vi "Run and Terminate Servos Arduino --LINX--.vi"(0 "Stop Button":bool, 1 "Angle 1":u16=500 min=500 max=2250, 2 "Angle 2":u16=500 min=500 max=2250, 3 "Angle 3":u16=500 min=500 max=2250, 4 "Angle 4":u16=500 min=500 max=2250, 5 "Error In":errorcluster, 6 "Motor 1":enum8{"B", "S", "E", "C"}(ring), 7 "LINX Resource":T2, 8 "Motor 2":enum8{"B", "S", "E", "C"}(ring)=enum."S", 10 "Motor 3":enum8{"B", "S", "E", "C"}(ring)=enum."E", 11 "No. of Motors":enum8{"1", "2", "3", "4"}(ring), 12 "Motor 4":enum8{"B", "S", "E", "C"}(ring)=enum."C", 13 "Board Type":T1(ring)) -> (9 "LINX Resource 2":T2, 14 "Stopped":T8, 19 "Error Out":errorcluster)   [LabVIEW 2015]
uses:
  Stopped Ind.ctl
  <vilib>/MakerHub/LINX/Private/Type Defs/LINX Ref.ctl
  <vilib>/MakerHub/LINX/Private/Type Defs/Platform.ctl
  <vilib>/MakerHub/LINX/Private/Type Defs/Interface.ctl
  <vilib>/MakerHub/LINX/Private/Device/Type Defs/LINX Device Config.ctl
  <vilib>/MakerHub/LINX/Private/Device/Type Defs/TCP Config.ctl
  <vilib>/MakerHub/LINX/Private/Device/Type Defs/Channels.ctl
  <vilib>/MakerHub/LINX/Public/Sensors/Motion/Servo/Servo Set Pulse Width N Channels.vi
  <vilib>/MakerHub/LINX/Public/Sensors/Motion/Servo/Servo Close N Channels.vi
  <vilib>/MakerHub/LINX/Public/Sensors/Motion/Servo/Servo.lvlib
  <vilib>/MakerHub/LINX/LMH-LINX.lvlib
  <vilib>/MakerHub/LINX/Private/Device/Device.lvlib
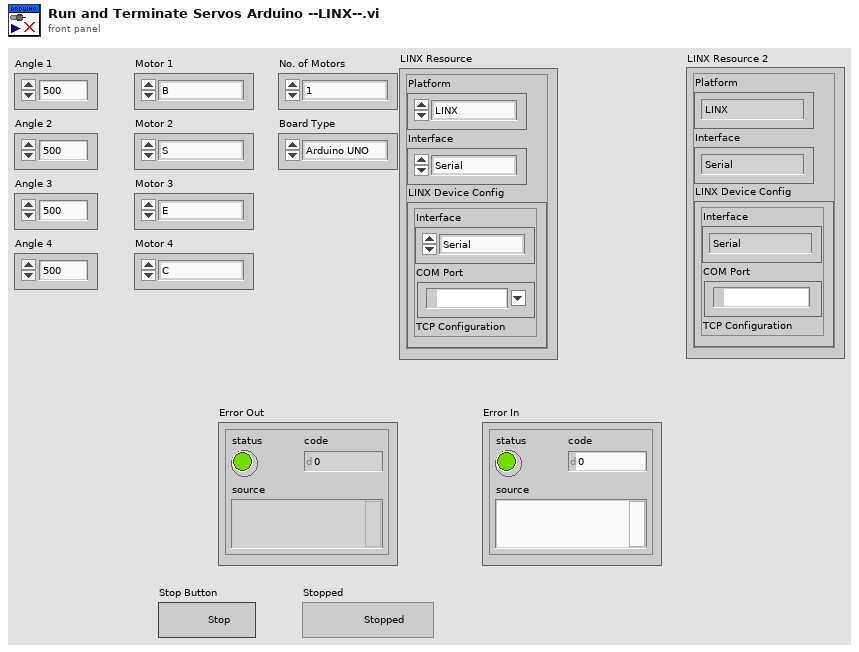
[diagram p1: front panel]
types:
  T1 = enum16{"Arduino UNO", "Arduino Leonardo", "Arduino Nano", "Arduino Pro Micro", "Arduino Mega 2560", "Arduino ADK"}
  T2 = typedef "LMH-LINX.lvlib/LINX Ref.ctl" = cluster{"Platform":T3, "Interface":T4, "LINX Device Config":T5}
  T3 = typedef "LMH-LINX.lvlib/Platform.ctl" = enum16{"LINX", "myRIO"}
  T4 = typedef "LMH-LINX.lvlib/Interface.ctl" = enum16{"Serial", "TCP"}
  T5 = typedef "LMH-LINX.lvlib/Device.lvlib/LINX Device Config.ctl" = cluster{"Interface":T4, "COM Port":refnum<visa-resource-name>, "TCP Configuration":T6, "Device Family":u8, "Device ID":u8, "Device Name":string, "TCP Ref":refnum<k5>, "Channels":T7}
  T6 = typedef "LMH-LINX.lvlib/Device.lvlib/TCP Config.ctl" = cluster{"IP Address":string, "Port":u16}
  T7 = typedef "LMH-LINX.lvlib/Channels.ctl" = cluster{"DI":u8[], "DO":u8[], "AI":u8[], "AO":u8[], "PWM":u8[], "QE":u8[], "UART":u8[], "I2C 2":u8[], "SPI":u8[], "CAN":u8[], "Servo":u8[], "AI Ref (V)":dbl, "AO Ref (V)":dbl, "AO Resolution (Bits)":u8}
  T8 = typedef "Stopped Ind.ctl" = bool
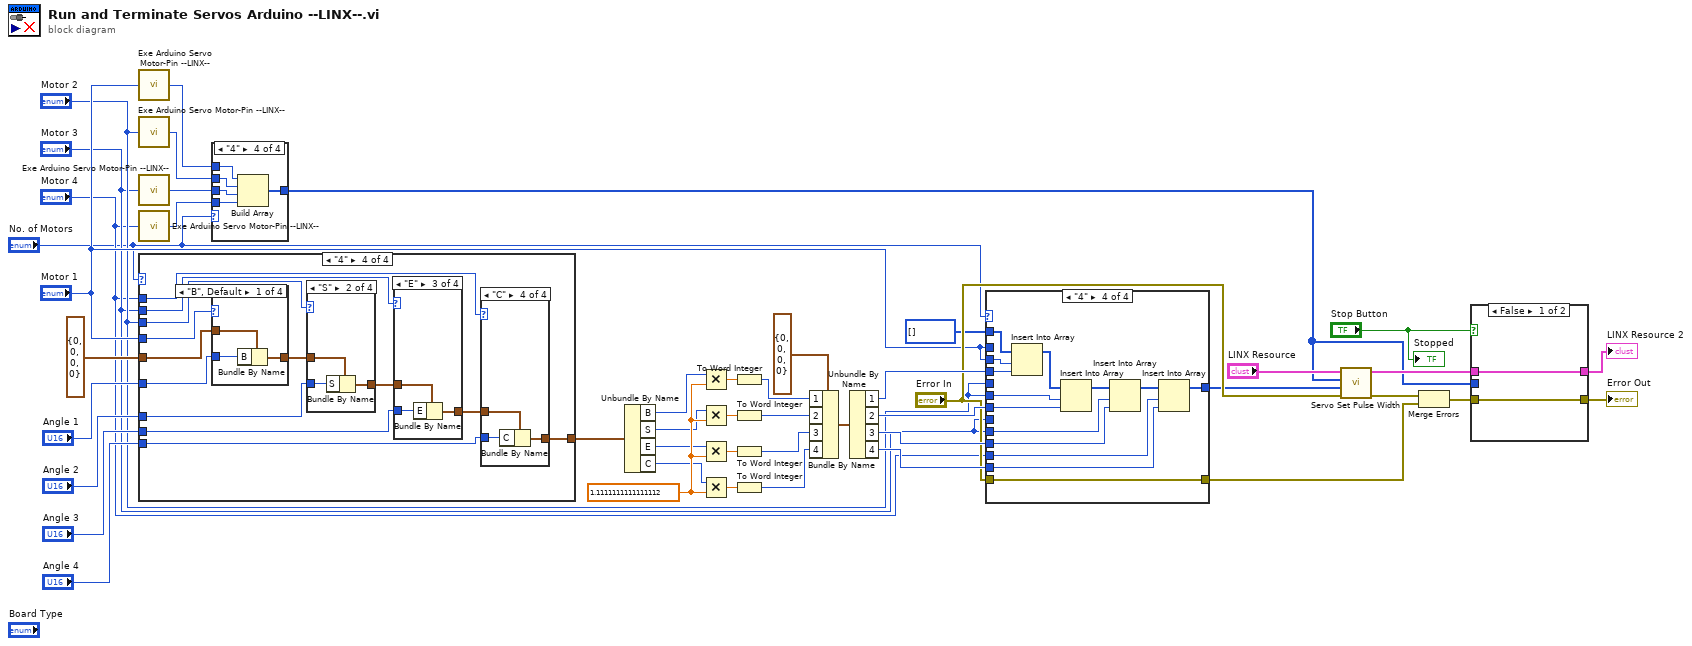
[diagram p0: block diagram]
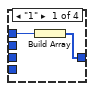
[diagram p2: hidden frame]
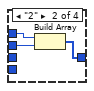
[diagram p3: hidden frame]
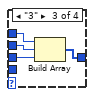
[diagram p4: hidden frame]
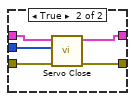
[diagram p5: hidden frame]
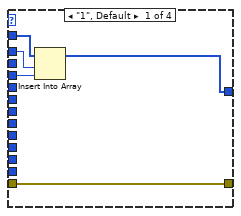
[diagram p6: hidden frame]
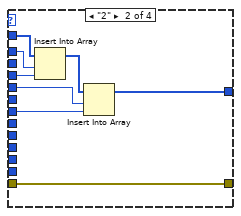
[diagram p7: hidden frame]
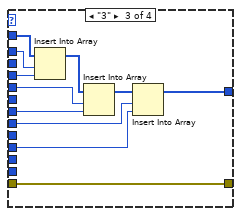
[diagram p8: hidden frame]
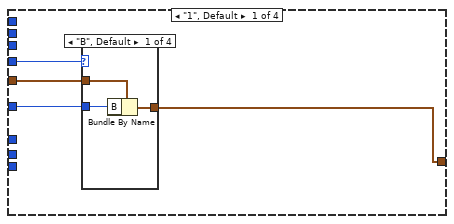
[diagram p9: hidden frame]
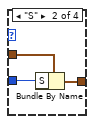
[diagram p10: hidden frame]
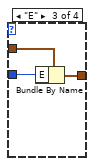
[diagram p11: hidden frame]
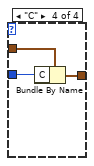
[diagram p12: hidden frame]
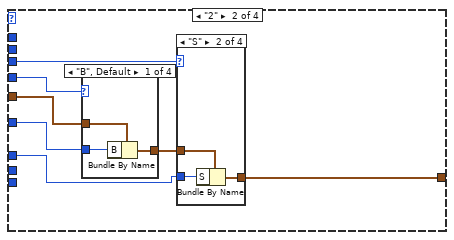
[diagram p13: hidden frame]
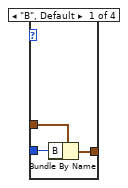
[diagram p14: hidden frame]
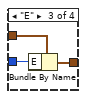
[diagram p15: hidden frame]
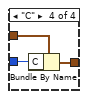
[diagram p16: hidden frame]
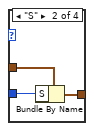
[diagram p17: hidden frame]
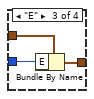
[diagram p18: hidden frame]
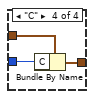
[diagram p19: hidden frame]
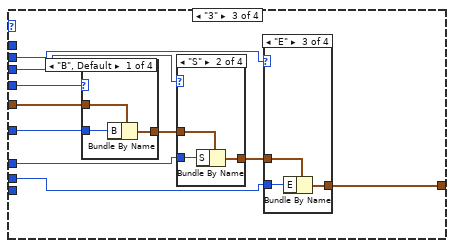
[diagram p20: hidden frame]
diagram:
  w36 = 1.1111111111111112 ("y")
  n1 = call "Exe Arduino Servo Motor-Pin --LINX--.vi"("Motor Name"="Motor 1") -> ("Pin"=w11:u8)
  n2 = call "Exe Arduino Servo Motor-Pin --LINX--.vi"("Motor Name"="Motor 2") -> ("Pin"=w9:u8)
  n3 = call "Exe Arduino Servo Motor-Pin --LINX--.vi"("Motor Name"="Motor 3") -> ("Pin"=w7:u8)
  n4 = call "Exe Arduino Servo Motor-Pin --LINX--.vi"("Motor Name"="Motor 4") -> ("Pin"=w6:u8)
  n5 = case shown="\"4\"" "No. of Motors" {
    tunnel: "Motor 1" -> [w50 w64 w99 w147]
    tunnel: "Motor 3" -> [_ _ w94 w145]
    tunnel: "Motor 4" -> [_ _ _ w144]
    tunnel: "Motor 2" -> [_ w63 w98 w146]
    tunnel: "Angle 4" -> [_ _ _ w140]
    tunnel: "Angle 2" -> [_ w66 w96 w142]
    tunnel: "Angle 3" -> [_ _ w95 w141]
    tunnel: "Angle 1" -> [w48 w67 w97 w143]
    tunnel: cluster{"B":i16, "S":i16, "E":i16, "C":i16} {"B"=0, "S"=0, "E"=0, "C"=0} ("Servos") -> [w49 w69 w101 w148]
    tunnel: [w47 w68 w102 w149] -> w41
    frame "1", Default {
      n6 = case shown="\"B\", Default" w50 {
        tunnel: w49 -> [w53 w56 w59 w61]
        tunnel: w48 -> [w51 w55 w57 w60]
        tunnel: [w52 w54 w58 w62] -> w47
        frame "B", Default {
          n7 = Bundle By Name(cluster=w53, "B"=w51) -> (w52:cluster{"B":i16, "S":i16, "E":i16, "C":i16})
        }
        frame "S" {
          n8 = Bundle By Name(cluster=w56, "S"=w55) -> (w54:cluster{"B":i16, "S":i16, "E":i16, "C":i16})
        }
        frame "E" {
          n9 = Bundle By Name(cluster=w59, "E"=w57) -> (w58:cluster{"B":i16, "S":i16, "E":i16, "C":i16})
        }
        frame "C" {
          n10 = Bundle By Name(cluster=w61, "C"=w60) -> (w62:cluster{"B":i16, "S":i16, "E":i16, "C":i16})
        }
      }
    }
    frame "2" {
      n11 = case shown="\"B\", Default" w64 {
        tunnel: w69 -> [w84 w87 w90 w93]
        tunnel: w67 -> [w82 w86 w88 w92]
        tunnel: [w83 w85 w89 w91] -> w65
        frame "B", Default {
          n12 = Bundle By Name(cluster=w84, "B"=w82) -> (w83:cluster{"B":i16, "S":i16, "E":i16, "C":i16})
        }
        frame "S" {
          n13 = Bundle By Name(cluster=w87, "S"=w86) -> (w85:cluster{"B":i16, "S":i16, "E":i16, "C":i16})
        }
        frame "E" {
          n14 = Bundle By Name(cluster=w90, "E"=w88) -> (w89:cluster{"B":i16, "S":i16, "E":i16, "C":i16})
        }
        frame "C" {
          n15 = Bundle By Name(cluster=w93, "C"=w92) -> (w91:cluster{"B":i16, "S":i16, "E":i16, "C":i16})
        }
      }
      n16 = case shown="\"S\"" w63 {
        tunnel: w65 -> [w72 w75 w78 w80]
        tunnel: w66 -> [w70 w74 w76 w79]
        tunnel: [w71 w73 w77 w81] -> w68
        frame "B", Default {
          n17 = Bundle By Name(cluster=w72, "B"=w70) -> (w71:cluster{"B":i16, "S":i16, "E":i16, "C":i16})
        }
        frame "S" {
          n18 = Bundle By Name(cluster=w75, "S"=w74) -> (w73:cluster{"B":i16, "S":i16, "E":i16, "C":i16})
        }
        frame "E" {
          n19 = Bundle By Name(cluster=w78, "E"=w76) -> (w77:cluster{"B":i16, "S":i16, "E":i16, "C":i16})
        }
        frame "C" {
          n20 = Bundle By Name(cluster=w80, "C"=w79) -> (w81:cluster{"B":i16, "S":i16, "E":i16, "C":i16})
        }
      }
    }
    frame "3" {
      n21 = case shown="\"B\", Default" w99 {
        tunnel: w101 -> [w106 w109 w112 w115]
        tunnel: w97 -> [w104 w108 w110 w114]
        tunnel: [w105 w107 w111 w113] -> w100
        frame "B", Default {
          n22 = Bundle By Name(cluster=w106, "B"=w104) -> (w105:cluster{"B":i16, "S":i16, "E":i16, "C":i16})
        }
        frame "S" {
          n23 = Bundle By Name(cluster=w109, "S"=w108) -> (w107:cluster{"B":i16, "S":i16, "E":i16, "C":i16})
        }
        frame "E" {
          n24 = Bundle By Name(cluster=w112, "E"=w110) -> (w111:cluster{"B":i16, "S":i16, "E":i16, "C":i16})
        }
        frame "C" {
          n25 = Bundle By Name(cluster=w115, "C"=w114) -> (w113:cluster{"B":i16, "S":i16, "E":i16, "C":i16})
        }
      }
      n26 = case shown="\"S\"" w98 {
        tunnel: w100 -> [w130 w133 w136 w138]
        tunnel: w96 -> [w128 w132 w134 w137]
        tunnel: [w129 w131 w135 w139] -> w103
        frame "B", Default {
          n27 = Bundle By Name(cluster=w130, "B"=w128) -> (w129:cluster{"B":i16, "S":i16, "E":i16, "C":i16})
        }
        frame "S" {
          n28 = Bundle By Name(cluster=w133, "S"=w132) -> (w131:cluster{"B":i16, "S":i16, "E":i16, "C":i16})
        }
        frame "E" {
          n29 = Bundle By Name(cluster=w136, "E"=w134) -> (w135:cluster{"B":i16, "S":i16, "E":i16, "C":i16})
        }
        frame "C" {
          n30 = Bundle By Name(cluster=w138, "C"=w137) -> (w139:cluster{"B":i16, "S":i16, "E":i16, "C":i16})
        }
      }
      n31 = case shown="\"E\"" w94 {
        tunnel: w103 -> [w118 w121 w124 w126]
        tunnel: [w117 w120 w123 w127] -> w102
        tunnel: w95 -> [w116 w119 w122 w125]
        frame "B", Default {
          n32 = Bundle By Name(cluster=w118, "B"=w116) -> (w117:cluster{"B":i16, "S":i16, "E":i16, "C":i16})
        }
        frame "S" {
          n33 = Bundle By Name(cluster=w121, "S"=w119) -> (w120:cluster{"B":i16, "S":i16, "E":i16, "C":i16})
        }
        frame "E" {
          n34 = Bundle By Name(cluster=w124, "E"=w122) -> (w123:cluster{"B":i16, "S":i16, "E":i16, "C":i16})
        }
        frame "C" {
          n35 = Bundle By Name(cluster=w126, "C"=w125) -> (w127:cluster{"B":i16, "S":i16, "E":i16, "C":i16})
        }
      }
    }
    frame "4" {
      n36 = case shown="\"B\", Default" w147 {
        tunnel: w148 -> [w155 w158 w161 w163]
        tunnel: w143 -> [w153 w157 w159 w162]
        tunnel: [w154 w156 w160 w164] -> w152
        frame "B", Default {
          n37 = Bundle By Name(cluster=w155, "B"=w153) -> (w154:cluster{"B":i16, "S":i16, "E":i16, "C":i16})
        }
        frame "S" {
          n38 = Bundle By Name(cluster=w158, "S"=w157) -> (w156:cluster{"B":i16, "S":i16, "E":i16, "C":i16})
        }
        frame "E" {
          n39 = Bundle By Name(cluster=w161, "E"=w159) -> (w160:cluster{"B":i16, "S":i16, "E":i16, "C":i16})
        }
        frame "C" {
          n40 = Bundle By Name(cluster=w163, "C"=w162) -> (w164:cluster{"B":i16, "S":i16, "E":i16, "C":i16})
        }
      }
      n41 = case shown="\"S\"" w146 {
        tunnel: w152 -> [w179 w182 w185 w187]
        tunnel: w142 -> [w177 w181 w183 w186]
        tunnel: [w178 w180 w184 w188] -> w151
        frame "B", Default {
          n42 = Bundle By Name(cluster=w179, "B"=w177) -> (w178:cluster{"B":i16, "S":i16, "E":i16, "C":i16})
        }
        frame "S" {
          n43 = Bundle By Name(cluster=w182, "S"=w181) -> (w180:cluster{"B":i16, "S":i16, "E":i16, "C":i16})
        }
        frame "E" {
          n44 = Bundle By Name(cluster=w185, "E"=w183) -> (w184:cluster{"B":i16, "S":i16, "E":i16, "C":i16})
        }
        frame "C" {
          n45 = Bundle By Name(cluster=w187, "C"=w186) -> (w188:cluster{"B":i16, "S":i16, "E":i16, "C":i16})
        }
      }
      n46 = case shown="\"E\"" w145 {
        tunnel: w151 -> [w191 w194 w197 w199]
        tunnel: w141 -> [w189 w193 w195 w198]
        tunnel: [w190 w192 w196 w200] -> w150
        frame "B", Default {
          n47 = Bundle By Name(cluster=w191, "B"=w189) -> (w190:cluster{"B":i16, "S":i16, "E":i16, "C":i16})
        }
        frame "S" {
          n48 = Bundle By Name(cluster=w194, "S"=w193) -> (w192:cluster{"B":i16, "S":i16, "E":i16, "C":i16})
        }
        frame "E" {
          n49 = Bundle By Name(cluster=w197, "E"=w195) -> (w196:cluster{"B":i16, "S":i16, "E":i16, "C":i16})
        }
        frame "C" {
          n50 = Bundle By Name(cluster=w199, "C"=w198) -> (w200:cluster{"B":i16, "S":i16, "E":i16, "C":i16})
        }
      }
      n51 = case shown="\"C\"" w144 {
        tunnel: w150 -> [w167 w170 w173 w175]
        tunnel: w140 -> [w165 w169 w171 w174]
        tunnel: [w166 w168 w172 w176] -> w149
        frame "B", Default {
          n52 = Bundle By Name(cluster=w167, "B"=w165) -> (w166:cluster{"B":i16, "S":i16, "E":i16, "C":i16})
        }
        frame "S" {
          n53 = Bundle By Name(cluster=w170, "S"=w169) -> (w168:cluster{"B":i16, "S":i16, "E":i16, "C":i16})
        }
        frame "E" {
          n54 = Bundle By Name(cluster=w173, "E"=w171) -> (w172:cluster{"B":i16, "S":i16, "E":i16, "C":i16})
        }
        frame "C" {
          n55 = Bundle By Name(cluster=w175, "C"=w174) -> (w176:cluster{"B":i16, "S":i16, "E":i16, "C":i16})
        }
      }
    }
  }
  n56 = case shown="\"4\"" "No. of Motors" {
    tunnel: [w201 w203 w208 w214] -> w14
    tunnel: w11 -> [w202 w205 w209 w213]
    tunnel: w9 -> [_ w204 w207 w212]
    tunnel: w7 -> [_ _ w206 w211]
    tunnel: w6 -> [_ _ _ w210]
    frame "1" {
      n57 = Build Array(w202) -> (w201:u8[])
    }
    frame "2" {
      n58 = Build Array(w205, w204) -> (w203:u8[])
    }
    frame "3" {
      n59 = Build Array(w209, w207, w206) -> (w208:u8[])
    }
    frame "4" {
      n60 = Build Array(w213, w212, w211, w210) -> (w214:u8[])
    }
  }
  n61 = Unbundle By Name(w41) -> ("B"=w39:i16, "S"=w29:i16, "E"=w28:i16, "C"=w27:i16)
  n62 = Multiply(x=w39, y=w36) -> (x*y=w37:dbl)
  n63 = Multiply(x=w29, y=w36) -> (x*y=w30:dbl)
  n64 = Multiply(x=w28, y=w36) -> (x*y=w33:dbl)
  n65 = Multiply(x=w27, y=w36) -> (x*y=w31:dbl)
  n66 = To Word Integer(number=w37) -> (16bit integer=w38:i16)
  n67 = To Word Integer(number=w30) -> (16bit integer=w34:i16)
  n68 = To Word Integer(number=w33) -> (16bit integer=w32:i16)
  n69 = To Word Integer(number=w31) -> (16bit integer=w35:i16)
  n70 = Bundle By Name(cluster=cluster{"1":i16, "2":i16, "3":i16, "4":i16} {"1"=0, "2"=0, "3"=0, "4"=0} ("Servo DC"), "1"=w38, "2"=w34, "3"=w32, "4"=w35) -> (w26:cluster{"1":i16, "2":i16, "3":i16, "4":i16})
  n71 = Unbundle By Name(w26) -> ("1"=w25:i16, "2"=w24:i16, "3"=w23:i16, "4"=w22:i16)
  n72 = case shown="\"4\"" "No. of Motors" {
    tunnel: "Motor 1" -> [w218 w224 w231 _]
    tunnel: "Motor 2" -> [_ w225 w233 _]
    tunnel: "Motor 3" -> [_ _ w235 _]
    tunnel: "Motor 4" -> [_ _ _ w245]
    tunnel: "Motor 3" -> [_ _ _ w246]
    tunnel: "Motor 2" -> [_ _ _ w247]
    tunnel: "Motor 1" -> [_ _ _ w248]
    tunnel: w25 -> [w217 w223 w230 w242]
    tunnel: w24 -> [_ w222 w232 w241]
    tunnel: w23 -> [_ _ w234 w240]
    tunnel: w22 -> [_ _ _ w239]
    tunnel: [w219 w227 w238 w252] -> w1
    tunnel: "Error In" -> [w219 w227 w238 w252]
    tunnel: u16[] [] ("Pulse Widths (uS)") -> [w216 w221 w229 w244]
    tunnel: [w215 w220 w228 w243] -> w16
    frame "1", Default {
      n73 = Insert Into Array(array=w216, index=w218, new element=w217) -> (w215:u16[])
    }
    frame "2" {
      n74 = Insert Into Array(array=w221, index=w224, new element=w223) -> (w226:u16[])
      n75 = Insert Into Array(array=w226, index=w225, new element=w222) -> (w220:u16[])
    }
    frame "3" {
      n76 = Insert Into Array(array=w229, index=w231, new element=w230) -> (w237:u16[])
      n77 = Insert Into Array(array=w237, index=w233, new element=w232) -> (w236:u16[])
      n78 = Insert Into Array(array=w236, index=w235, new element=w234) -> (w228:u16[])
    }
    frame "4" {
      n79 = Insert Into Array(array=w244, index=w248, new element=w242) -> (w249:u16[])
      n80 = Insert Into Array(array=w249, index=w247, new element=w241) -> (w250:u16[])
      n81 = Insert Into Array(array=w250, index=w246, new element=w240) -> (w251:u16[])
      n82 = Insert Into Array(array=w251, index=w245, new element=w239) -> (w243:u16[])
    }
  }
  n83 = call-poly <vilib>:"Servo Set Pulse Width.vi"("Error In"="Error In", "Pulse Widths (uS)"=w16, "Servo Channels"=w14, "LINX Resource"="LINX Resource") -> ("Error Out"=w2:errorcluster, "LINX Resource"=w15:T2)  [unwired: 6 in]
  n84 = Merge Errors(w2, w1) -> (w3:errorcluster)
  n85 = case shown="False" "Stop Button" {
    tunnel: w3 -> [w254 w259]
    tunnel: [w254 w258] -> w21
    tunnel: w15 -> [w253 w257]
    tunnel: w14 -> [_ w256]
    tunnel: [w253 w255] -> w13
    frame False {
    }
    frame True {
      n86 = call-poly <vilib>:"Servo Close.vi"("Error In"=w259, "Servo Channels"=w256, "LINX Resource"=w257) -> ("Error Out"=w258:errorcluster, "LINX Resource"=w255:T2)  [unwired: 7 in]
    }
  }
  "Error Out" <- w21
  "LINX Resource 2" <- w13
  "Stopped" <- "Stop Button"
